vi "RTM.vi"() -> ()   [LabVIEW 2017]
uses:
  <vilib>/Simulation/Scripting/Companion Diagram/SimConfigNode/SimParams.ctl
  <vilib>/Simulation/Scripting/Companion Diagram/SimConfigNode/_simSolvers.ctl
  <vilib>/Simulation/Implementation/Shared/SIMSCR Execution Mode.ctl
  <vilib>/Simulation/Param Hierarchy/Typedefs/SIMPH Param Control Actions.ctl
  <vilib>/Simulation/Implementation/Shared/SIM limit type.ctl
  <vilib>/Simulation/Implementation/Shared/NILVSim_ParamChanged.vi
  <vilib>/Simulation/Implementation/Shared/NILVSIM_BeginStep.vi
  <vilib>/Simulation/SignalDisplay/Implementation/NILVSim Time Waveform.llb/SIM Time Waveform (vector).vi
  <vilib>/Simulation/ContinuousLinear/Implementation/NILVSim Derivative.llb/SIM derivative (scalar).vi
  <vilib>/Simulation/SignalDisplay/Implementation/NILVSim Time Waveform.llb/SIM Time Waveform (scalar).vi
  <vilib>/Simulation/ContinuousLinear/Implementation/NILVSim Integrator new.llb/SIM Integrator distributor (scalar).vi
  <vilib>/Simulation/SignalDisplay/Implementation/NILVSim Buffer XY Graph.llb/SIM Buffer XY Graph (scalar).vi
  <vilib>/Simulation/ContinuousLinear/Implementation/NILVSim Integrator new.llb/SIM Integrator collector (scalar).vi
  <vilib>/Simulation/Implementation/Shared/NILVSim_Manager.vi
  <vilib>/Utility/error.llb/Clear Errors.vi
  <vilib>/Simulation/Implementation/Shared/NILVSim_FinalizeModel.vi
  <vilib>/Simulation/SignalDisplay/Implementation/NILVSim Buffer XY Graph.llb/NILVSim Buffer XY Graph (core).vi
  <vilib>/Simulation/Implementation/Shared/SIM manage modulo counter.vi
  <vilib>/Simulation/Implementation/Shared/SIM Circular Buffer.llb/SIM CircBuf remove oldest.vi
  <vilib>/Simulation/Implementation/Shared/SIM Circular Buffer.llb/SIM circular buffer insert.vi
  <vilib>/Simulation/Implementation/Shared/SIM Unbundle Sim Info.vi
  <vilib>/Simulation/Implementation/Shared/NILVSim_Initialize.vi
  <vilib>/addons/control/pid/pid.llb/PID.vi
  <vilib>/addons/control/pid/pid.llb/PID (DBL).vi
  <vilib>/Simulation/Implementation/Shared/SIM Circular Buffer.llb/SIM circular buffer create.vi
  <vilib>/Simulation/Implementation/Shared/SIM Circular Buffer.llb/SIM circular buffer ordered array.vi
  <vilib>/Simulation/Utility/Implementation/NILVSim Get Time and IsAcceptedStep.vi
  Test.vi
  Model.vi
  <vilib>/Simulation/Implementation/Shared/SIMSH Read Queue.vi
  <vilib>/Simulation/Implementation/Shared/NILVSim_GetModelError.vi
  <vilib>/Simulation/Implementation/Shared/SIM Bundle Sim Info.vi
  <vilib>/Simulation/Scripting/Companion Diagram/SimConfigNode/SimDog.xnode
  <vilib>/Simulation/Implementation/XNodeFramework/SimXNode/SimX.xnode
  <vilib>/Simulation/ContinuousLinear/Implementation/NILVSim Integrator new.llb/SIM Integrator (scalar).vi
  <vilib>/addons/control/pid/NI_PID_pid.lvlib
  <vilib>/Simulation/Implementation/Shared/NI_SIM_Implementation.lvlib
panel:
  out "error":dbl
  in  "PID gains":T1={"proportional gain (Kc)"=0.5, "integral time (Ti, min)"=5.0, "derivative time (Td, min)"=1.5000000000000002}
  out "Control Signal":waveform(dbl)(graph)={"t0"=timestamp(9343.2 s since 1904-01-01), "dt"=1.0, "Y"=[0.2633720690985406]}
  in  "Theta (Orientation)":dbl(knob) scale=0.0..359.0 scale format="%#_2f"
  out "V":dbl
  out "Vx":dbl
  out "Vy":dbl
  out "wr (rad/sec)":dbl
  out "WL (RPM)":dbl(knob) scale=0.0..200.0
  out "WR (RPM)":dbl(knob) scale=0.0..200.0
  out "wl (rad/sec)":dbl
  in  "V Setpoint":dbl(slide) scale=0.0..10.0
  out "Y (meter)":dbl
  out "X (meter)":dbl
  out "w":waveform(dbl)(graph)={"t0"=timestamp(9343.2 s since 1904-01-01), "dt"=1.0, "Y"=[0.2633720690985406]}
  out "Linear Speed":waveform(dbl)[](graph)
  out "Chart Degree":dbl(graph)
  out "XY (km)":cluster{"X":dbl, "Y":dbl}[](graph)
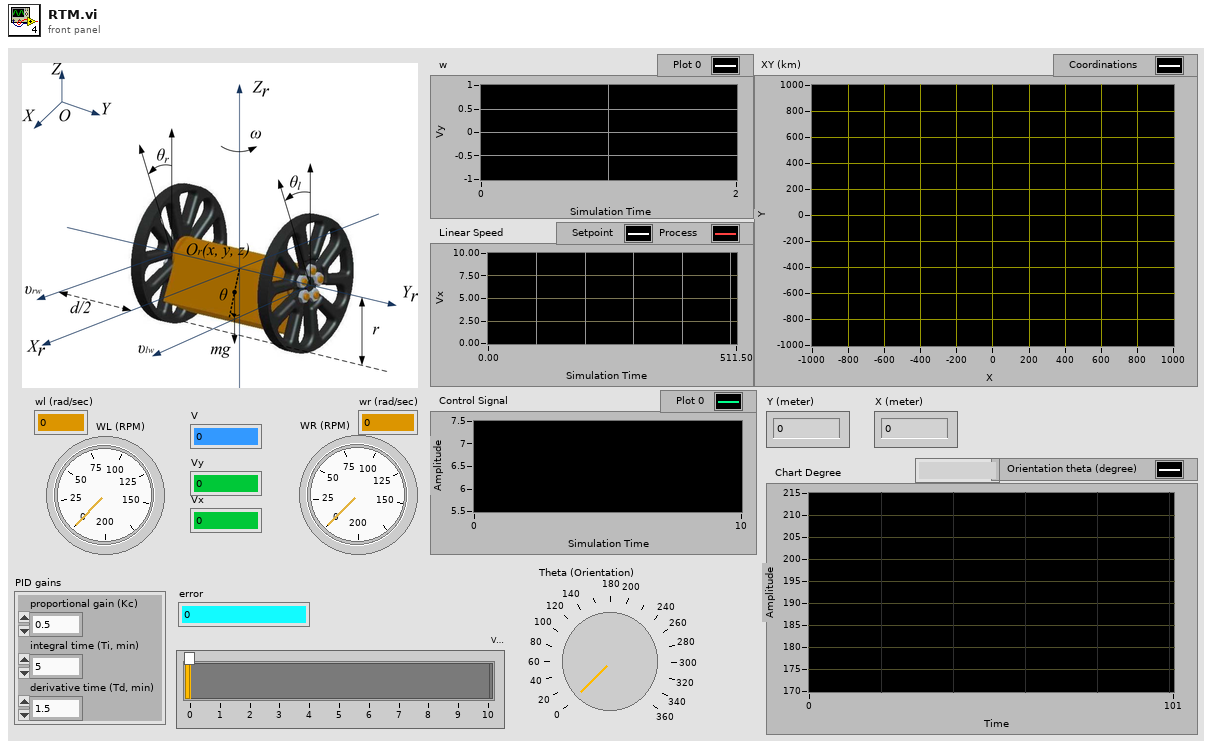
[diagram p1: front panel]
types:
  T1 = cluster{"proportional gain (Kc)":dbl, "integral time (Ti, min)":dbl, "derivative time (Td, min)":dbl}
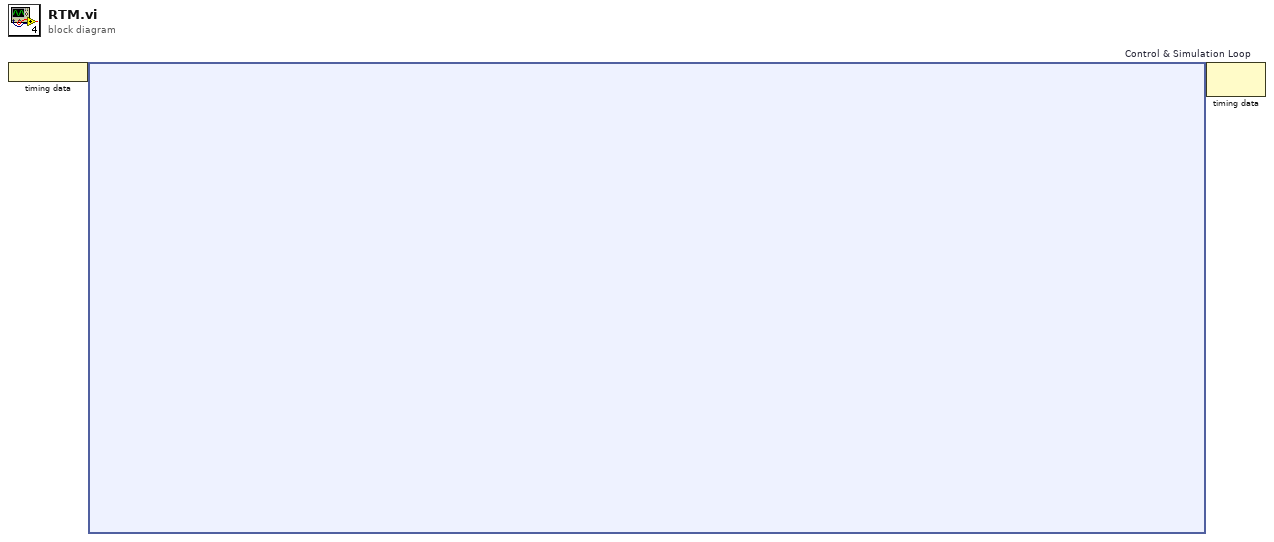
[diagram p0: block diagram]
diagram:
  n1 = node-c288() -> (w2:variant)
  n2 = node-c254 "Control & Simulation Loop"(w2) -> (w1:variant)
  n3 = node-c288(w1) -> ()  [unwired: 1 out]
